vi "Read JSON Config.vi"(8 "error in":errorcluster, 11 "object in":refnum<class "Configuration Base.lvclass">) -> (0 "error out":errorcluster, 2 "<JSON>Config":string, 3 "object out":refnum<class "Configuration Base.lvclass">)   [LabVIEW 2023, in "Configuration Base.lvlib" / "Configuration Base.lvclass"]
uses:
  Configuration Base.lvclass
  Configuration Base.lvclass/Configuration Base.ctl
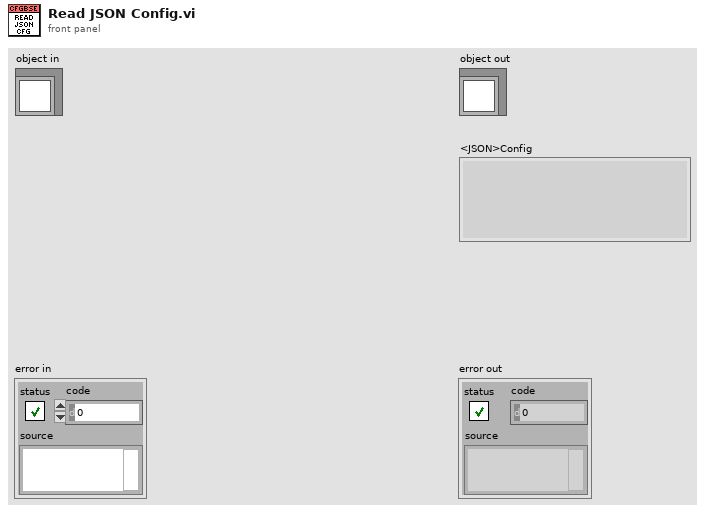
[diagram p1: front panel]
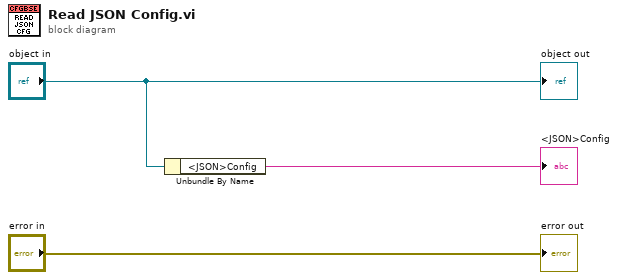
[diagram p0: block diagram]
diagram:
  n1 = Unbundle By Name("object in") -> ("<JSON>Config"=→"<JSON>Config":string)
  "error out" <- "error in"
  "object out" <- "object in"
